vi "Clear Specific Errors.vi"   [LabVIEW 2019, in "TSC Error.lvlib"]
doc: "This VI will clear a specific error code (or array of codes) if that is the error on the wire.\n\n<b>Code Developed By:</b>\nDaniel Coons\nTechnology Service Corporation\n1983 S Liberty Drive\nBloomington, IN 47403\nwww.tsc.com/atcs"
uses:
  TSC Error.lvlib
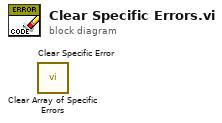
[diagram p0: block diagram]
diagram:
  n1 = call "Clear Array of Specific Errors.vi"() -> ()  [unwired: 11 in, 1 out]
  n2 = call "Clear Specific Error.vi"() -> ()  [unwired: 11 in, 1 out]
